vi "Unwind Turret.vi"(8 "error in (no error)":errorcluster, 10 "Unwind?":bool, 11 "Turret in":refnum<class "Turret.lvclass">) -> (0 "error out":errorcluster, 2 "Unwinding":bool, 3 "Turret out":refnum<class "Turret.lvclass">)   [LabVIEW 2019, in "Turret.lvlib" / "Turret.lvclass"]
uses:
  Turret.lvclass
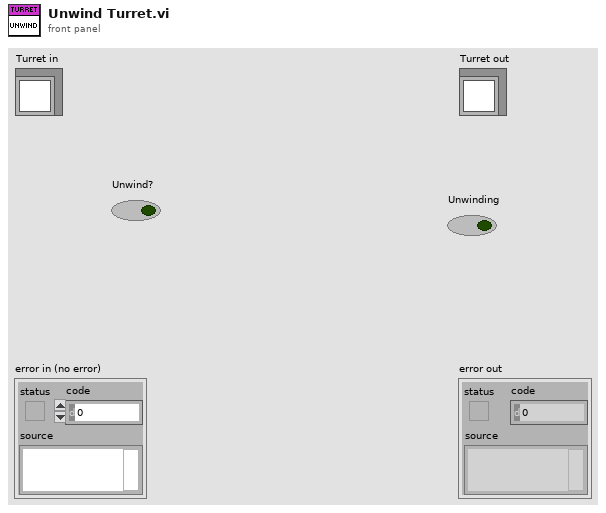
[diagram p1: front panel]
types:
  T1 = typedef "WPI_PotentiometerDevRef.ctl" = cluster{"DevStatus":errorcluster, "Analog Channel":T2, "Invert Output":bool}
  T2 = typedef "FPGA_AIChannel.ctl" = enum8{"AI 0", "AI 1", "AI 2", "AI 3", "AI MXP 0", "AI MXP 1", "AI MXP 2", "AI MXP 3", "Invalid"}
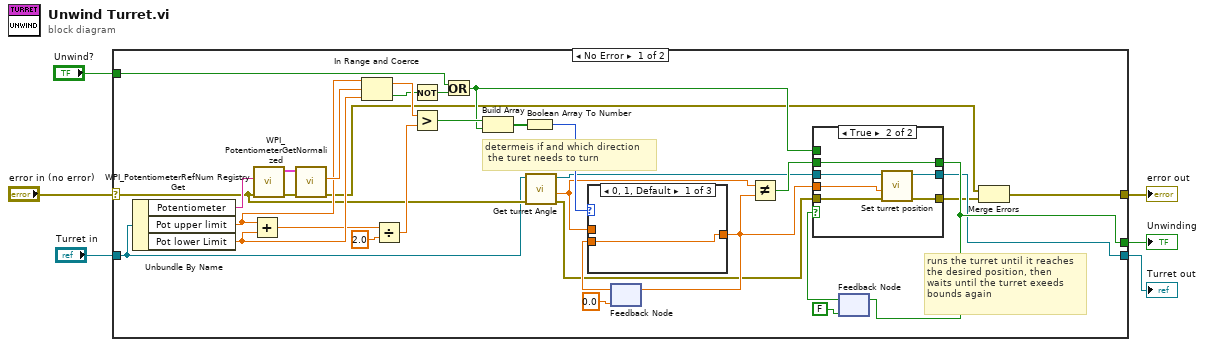
[diagram p0: block diagram]
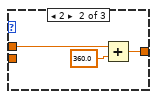
[diagram p3: hidden frame]
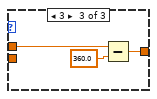
[diagram p4: hidden frame]
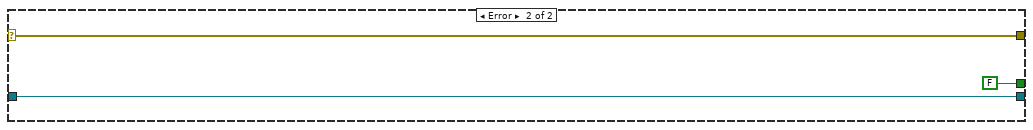
[diagram p5: hidden frame]
diagram:
  n1 = case shown="No Error" "error in (no error)" {
    selector: "error in (no error)" -> [w11 w58]
    tunnel: [w13 w58] -> w5
    tunnel: [w16 w57] -> w3
    tunnel: "Turret in" -> [w9 w57]
    tunnel: "Unwind?" -> [w26 _]
    tunnel: [w17 FALSE] -> w1
    frame No Error {
      # "runs the turret until it reaches \nthe desired position, then \nwaits until the turret exeeds \nbounds again"
      # "determeis if and which direction\n the turet needs to turn"
      n2 = Unbundle By Name(w9) -> ("Potentiometer"=w36:string, "Pot upper limit"=w29:dbl, "Pot lower Limit"=w35:dbl)
      n3 = Add(x=w29, y=w35) -> (x+y=w34:dbl)
      n4 = call <vilib>:"WPI_PotentiometerRefNum Registry Get.vi"("error in (no error)"=w11, "refnum name"=w36) -> ("error out"=w38:errorcluster, "PotDevRef"=w39:T1)  [unwired: 8 in]
      n5 = call <vilib>:"WPI_PotentiometerGetNormalized.vi"("error in"=w38, "PotDevRef"=w39) -> ("error out"=w14:errorcluster, "Normalized Value"=w37:dbl)  [unwired: 7 in, 1 out]
      n6 = In Range and Coerce(upper limit=w29, x=w37, lower limit=w35) -> (coerced(x)=w32:dbl, In Range?=w27:bool)
      n7 = Divide(x=w34, y=2.0) -> (x/y=w28:dbl)
      n8 = Not(x=w27) -> (.not. x?=w12:bool)
      n9 = Greater?(x=w32, y=w28) -> (0:w31:bool)
      n10 = Or(x=w26, y=w12) -> (x .or. y?=w21:bool)
      n11 = Build Array(w31, w21) -> (w30:bool[])
      n12 = Boolean Array To Number(Boolean array=w30) -> (number=w25:u32)
      n13 = call "Get turret Angle.vi"("error in (no error)"=w11, "Turret in"=w9) -> ("error out"=w10:errorcluster, "Turret Angle(deg)"=w7:dbl, "Turret out"=w8:refnum<class "Turret.lvclass">)  [unwired: 7 in]
      n14 = feedback #1(0.0) -> (w23:dbl)
      n15 = case shown="0, 1, Default" w25 {
        tunnel: [w49 w52 w55] -> w22
        tunnel: w23 -> [w49 _ _]
        tunnel: w7 -> [_ w51 w53]
        frame 0, 1, Default {
        }
        frame 2 {
          n16 = Add(x=w51, y=360.0) -> (x+y=w52:dbl)
        }
        frame 3 {
          n17 = Subtract(x=w53, y=360.0) -> (x-y=w55:dbl)
        }
      }
      n18 = feedback-in #1(w22) -> ()
      n19 = Not Equal?(x=w7, y=w22) -> (x != y?=w20:bool)
      n20 = feedback #2(FALSE) -> (w19:bool)
      n21 = case shown="True" w19 {
        tunnel: w22 -> [_ w47]
        tunnel: w21 -> [w42 _]
        tunnel: w20 -> [_ w48]
        tunnel: [w42 w48] -> w17
        tunnel: w8 -> [w40 w46]
        tunnel: [w40 w45] -> w16
        tunnel: w10 -> [w41 w44]
        tunnel: [w41 w43] -> w15
        frame False {
        }
        frame True {
          n22 = call "Set turret position.vi"("error in (no error)"=w44, "position(deg)"=w47, "Turret in"=w46) -> ("error out"=w43:errorcluster, "Turret out"=w45:refnum<class "Turret.lvclass">)  [unwired: 7 in]
        }
      }
      n23 = feedback-in #2(w17) -> ()
      n24 = Merge Errors(w14, w15) -> (w13:errorcluster)
    }
    frame Error {
    }
  }
  "error out" <- w5
  "Turret out" <- w3
  "Unwinding" <- w1
